vi "AG33XXX.ProcPeriodic.vi"(0 "i ref in":refnum<vi>, 3 "ms timeout (10000)":i32=10000, 5 "error in (no error)":errorcluster) -> (14 "i ref out":refnum<vi>, 17 "timed out":bool, 19 "error out":errorcluster)   [LabVIEW 2014, in "AG33XXX.lvlib"]
doc: "This method serves to periodically do things like reading values from the HW. Methods that should be executed periodically should be called from THIS method. Add code here."
uses:
  AG33XXX.lvlib
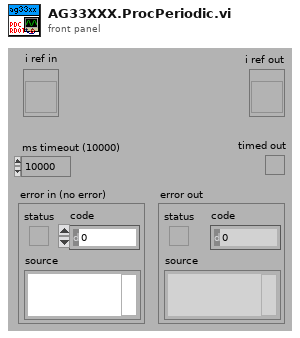
[diagram p1: front panel]
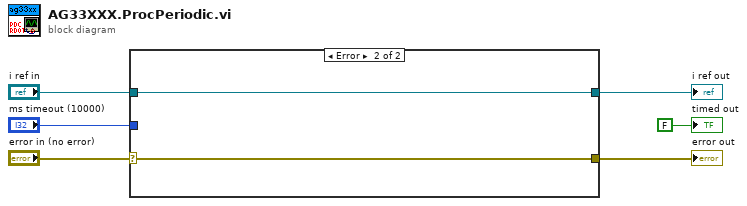
[diagram p0: block diagram]
diagram:
  n1 = case shown="Error" "error in (no error)" {
    selector: "error in (no error)" -> [w8 w9]
    tunnel: [w8 w9] -> w5
    tunnel: "i ref in" -> [w7 w10]
    tunnel: [w7 w10] -> w3
    tunnel: "ms timeout (10000)" -> [_ _]
    frame No Error {
      # "insert your code here"
    }
    frame Error {
    }
  }
  "error out" <- w5
  "i ref out" <- w3
  "timed out" <- FALSE ("timed out")
